vi "2. Calculate the distance traveled by the robot.vi"() -> ()   [LabVIEW 2020]
uses:
  <vilib>/robotics/Starter Kit/2.0/9632 Host Interface/NI_Robotics_Starter Kit Host_9632_2.0.lvclass
panel:
  in  "Servo Motor Value":dbl(slide) scale=-65.0..65.0
  in  "Distance":dbl(knob) scale=0.0..10.0
  in  "stop":bool
  out "Waveform Chart":cluster{"distance (m)":dbl, dbl, dbl}(graph)
  in  "Robot Velocity":dbl(slide) scale=0.0..0.3
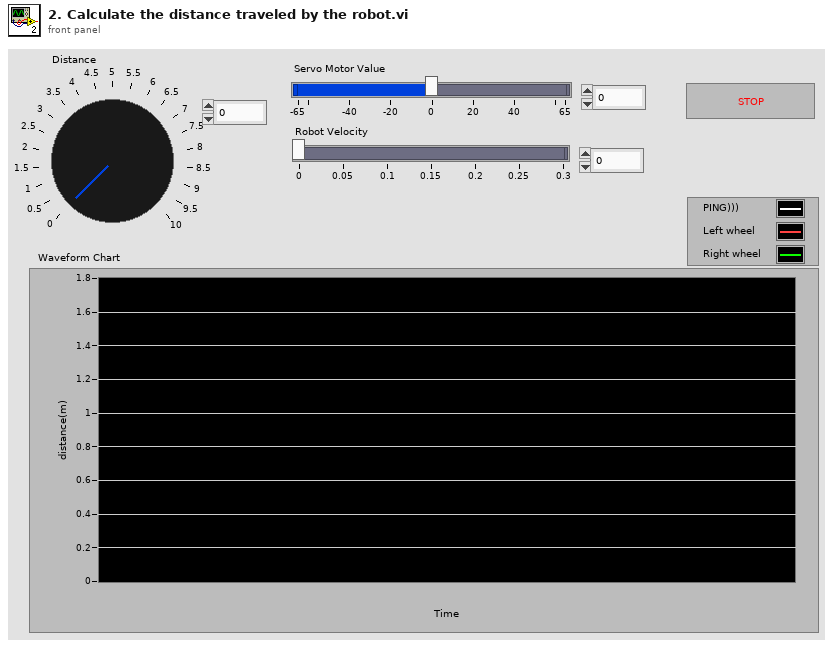
[diagram p1: front panel]
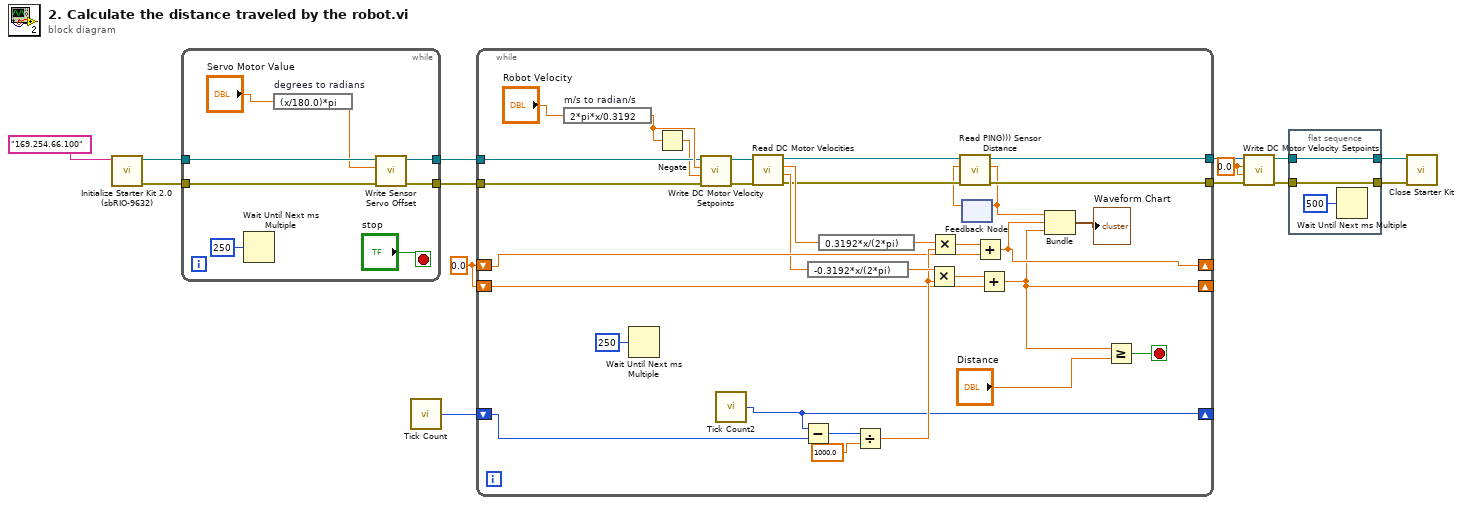
[diagram p0: block diagram]
diagram:
  w1 = 0.0
  w11 = 0.0 ("left motor ccw velocity (rad/s)")
  n1 = call <vilib>:"Initialize Starter Kit 2.0 (sbRIO-9632).vi"("IP address (\"\")"="169.254.66.100" ("IP address (\"\")")) -> ("error out"=w4:errorcluster, "FPGA starter kit host 2.0 out"=w6:refnum<class "NI_Robotics_Starter Kit Host_9632_2.0.lvclass">)  [unwired: 9 in]
  n2 = while {
    tunnel: w6 -> [w22]
    tunnel: [w20] -> w5
    tunnel: w4 -> [w21]
    tunnel: [w19] -> w3
    stop <- "stop" stop-if-true
    n3 = Wait Until Next ms Multiple(millisecond multiple=u32 250) -> ()  [unwired: 1 out]
    n4 = expression code="(x/180.0)*pi" "degrees to radians"("Servo Motor Value") -> (w16:dbl)
    n5 = call <vilib>:"Write Sensor Servo Offset.vi"("error in (no error)"=w21, "ccw offset angle (rad)"=w16, "starter kit host in"=w22) -> ("error out"=w19:errorcluster, "starter kit host out"=w20:refnum<class "NI_Robotics_Starter Kit Host_9632_2.0.lvclass">)  [unwired: 7 in]
  }
  n6 = call "Tick Count"() -> ("Tick Count(mSec)"=w2:u32)
  n7 = while {
    tunnel: w5 -> [w50]
    tunnel: w3 -> [w49]
    tunnel: [w27] -> w13
    tunnel: [w26] -> w12
    shift-right: [w35] -> _
    shift-left: w2 -> [w43]
    shift-right: [w39] -> _
    shift-left: w1 -> [w33]
    shift-right: [w38] -> _
    shift-left: w1 -> [w32]
    stop <- w41 stop-if-true
    n8 = expression code="2*pi*x/0.3192" "m/s to radian/s"("Robot Velocity") -> (w53:dbl)
    n9 = Wait Until Next ms Multiple(millisecond multiple=u32 250) -> ()  [unwired: 1 out]
    n10 = Negate(x=w53) -> (-x=w34:dbl)
    n11 = call <vilib>:"Write DC Motor Velocity Setpoints.vi"("error in (no error)"=w49, "right motor ccw velocity (rad/s)"=w34, "left motor ccw velocity (rad/s)"=w53, "starter kit host in"=w50) -> ("error out"=w52:errorcluster, "starter kit host out"=w51:refnum<class "NI_Robotics_Starter Kit Host_9632_2.0.lvclass">)  [unwired: 6 in]
    n12 = call "Tick Count2"() -> ("Tick Count(mSec)"=w35:u32)
    n13 = call <vilib>:"Read DC Motor Velocities.vi"("error in (no error)"=w52, "starter kit host in"=w51) -> ("error out"=w28:errorcluster, "right motor ccw velocity (rad/s)"=w31:dbl, "left motor ccw velocity (rad/s)"=w30:dbl, "starter kit host out"=w29:refnum<class "NI_Robotics_Starter Kit Host_9632_2.0.lvclass">)  [unwired: 6 in]
    n14 = Subtract(x=w35, y=w43) -> (x-y=w44:u32)
    n15 = expression code="-0.3192*x/(2*pi)" ("radian/s to RPM")(w31) -> (w46:dbl)
    n16 = expression code="0.3192*x/(2*pi)" ("radian/s to RPM")(w30) -> (w48:dbl)
    n17 = Divide(x=w44, y=1000.0) -> (x/y=w40:dbl)
    n18 = Multiply(x=w46, y=w40) -> (x*y=w45:dbl)
    n19 = Multiply(x=w48, y=w40) -> (x*y=w47:dbl)
    n20 = feedback #1() -> (w25:dbl)  [unwired: 1 in]
    n21 = call <vilib>:"Read PING))) Sensor Distance.vi"("error in (no error)"=w28, "default distance (NaN)"=w25, "starter kit host in"=w29) -> ("error out"=w26:errorcluster, "distance (m)"=w24:dbl, "starter kit host out"=w27:refnum<class "NI_Robotics_Starter Kit Host_9632_2.0.lvclass">)  [unwired: 5 in, 1 out]
    n22 = feedback-in #1(w24) -> ()
    n23 = Add(x=w47, y=w33) -> (x+y=w39:dbl)
    n24 = Add(x=w45, y=w32) -> (x+y=w38:dbl)
    n25 = Bundle("distance (m)"=w24, w39, w38) -> (→"Waveform Chart":cluster{"distance (m)":dbl, dbl, dbl})  [unwired: 1 in]
    n26 = Greater Or Equal?(x=w38, y="Distance") -> (x >= y?=w41:bool)
  }
  n27 = call <vilib>:"Write DC Motor Velocity Setpoints.vi"("error in (no error)"=w12, "right motor ccw velocity (rad/s)"=w11, "left motor ccw velocity (rad/s)"=w11, "starter kit host in"=w13) -> ("error out"=w9:errorcluster, "starter kit host out"=w10:refnum<class "NI_Robotics_Starter Kit Host_9632_2.0.lvclass">)  [unwired: 6 in]
  n28 = flat-sequence {
    tunnel: w10 -> [w57]
    tunnel: w9 -> [w56]
    tunnel: [w57] -> w8
    tunnel: [w56] -> w7
    frame #0 {
      n29 = Wait Until Next ms Multiple(millisecond multiple=u32 500) -> ()  [unwired: 1 out]
    }
  }
  n30 = call-dynamic "Close Starter Kit.vi"("error in (no error)"=w7, "starter kit host in"=w8) -> ()  [unwired: 9 in, 1 out]
